vi "Get Object by Ctl-Label.vi"(8 "error in":errorcluster, 10 "Ctl Label":string, 11 "Button Manager in":refnum<class "Button Manager.lvclass">) -> (0 "error out":errorcluster, 2 "Button Object":T1, 3 "Button Manager out":refnum<class "Button Manager.lvclass">)   [LabVIEW 2022 SP3, in "Navigation.lvlib" / "Button Manager.lvclass"]
doc: "____\nHAMPEL SOFTWARE ENGINEERING v2.6.0 (2023-12-19 10:54)"
uses:
  Button Manager.lvclass
  Top Control.ctl
  Sub Control.ctl
  Button Def.ctl
  Button Manager.lvclass/Button Manager.ctl
  <vilib>/Utility/error.llb/Error Cluster From Error Code.vi
  <vilib>/ErrorRing/Error Ring.xnode
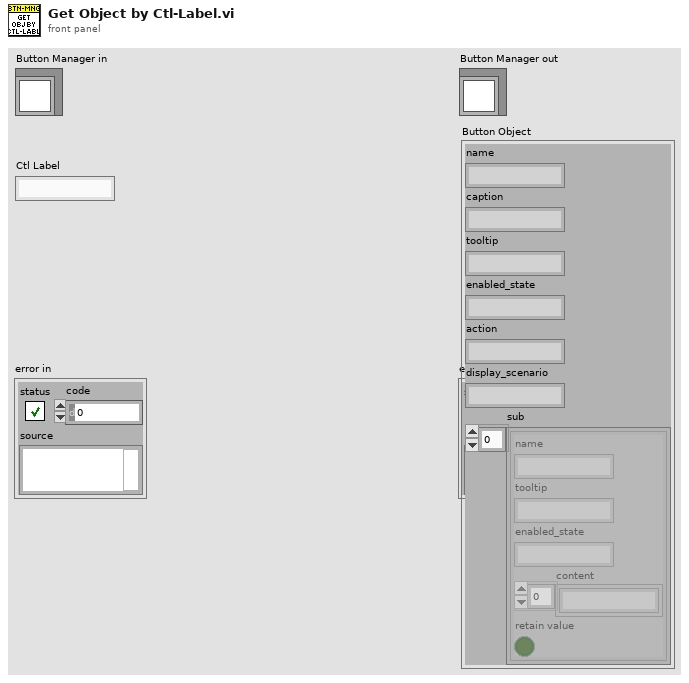
[diagram p1: front panel]
types:
  T1 = typedef "Navigation.lvlib/Button Manager.lvclass/Top Control.ctl" = cluster{"name":string, "caption":string, "tooltip":string, "enabled_state":string, "action":string, "display_scenario":string, "sub":T2[]}
  T2 = typedef "Navigation.lvlib/Button Manager.lvclass/Sub Control.ctl" = cluster{"name":string, "tooltip":string, "enabled_state":string, "content":string[], "retain value":bool}
  T3 = typedef "Navigation.lvlib/Button Manager.lvclass/Button Def.ctl" = cluster{"Top-Ctl Ref":refnum<vi>, "Sub-Ctl Ref":refnum<vi>, "Button Object":T1}
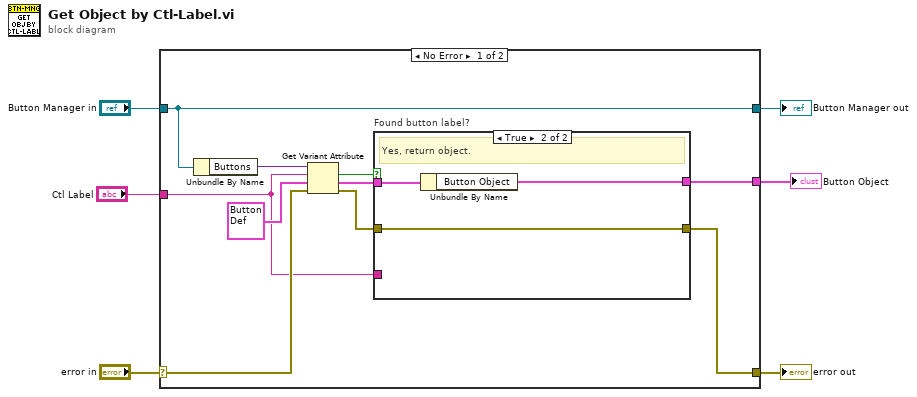
[diagram p0: block diagram]
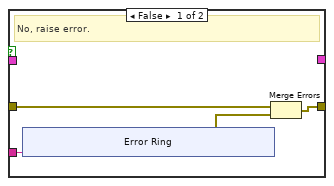
[diagram p2: hidden frame]
diagram:
  n1 = case shown="No Error" "error in" {
    selector: "error in" -> [w13 w32]
    tunnel: [w7 w32] -> w5
    tunnel: [w16 w31] -> w3
    tunnel: "Button Manager in" -> [w16 w31]
    tunnel: "Ctl Label" -> [w9 _]
    tunnel: [w8 _] -> w1
    frame No Error {
      n2 = Unbundle By Name(w16) -> ("Buttons"=w15:variant)
      n3 = Get Variant Attribute(Variant=w15, name=w9, default value (empty Variant)=T3 {"Top-Ctl Ref"=refnum, "Sub-Ctl Ref"=refnum, "Button Object"={"name"="", "caption"="", "tooltip"="", "enabled_state"="", "action"="", "display_scenario"="", "sub"=[]}} ("Button Def"), error in=w13) -> (found=w12:bool, value=w11:T3, error out=w10:errorcluster)  [unwired: 1 out]
      n4 = case "Found button label?" shown="True" w12 {
        tunnel: w11 -> [_ w30]
        tunnel: w10 -> [w18 w28]
        tunnel: [_ w29] -> w8
        tunnel: [w19 w28] -> w7
        tunnel: w9 -> [w17 _]
        frame False {
          # "No, raise error."
          n5 = xnode "Error Ring"("parameter 0"=w17) -> ("error out"=w20:errorcluster)
          n6 = Merge Errors(w18, w20) -> (w19:errorcluster)
        }
        frame True {
          # "Yes, return object."
          n7 = Unbundle By Name(w30) -> ("Button Object"=w29:T1)
        }
      }
    }
    frame Error {
    }
  }
  "error out" <- w5
  "Button Manager out" <- w3
  "Button Object" <- w1
